vi "TS Station Global Update UI.vi"(8 "error in (no error)":errorcluster, 11 "Auto UI in":refnum<class "Auto UI.lvclass">) -> (0 "error out":errorcluster, 3 "Auto UI out":refnum<class "Auto UI.lvclass">)   [LabVIEW 2023, in "GUI.lvlib" / "Auto UI.lvlib" / "Auto UI.lvclass"]
uses:
  Auto UI.lvclass
  Typdefs/Auto GUI/Test Info.ctl
  Typdefs/Auto GUI/Cycles and Mode.ctl
  Auto UI.lvclass/Auto UI.ctl
  GUI.lvlib
  HardwareAbstractionLayer_LVOOP/Database/Database.lvclass
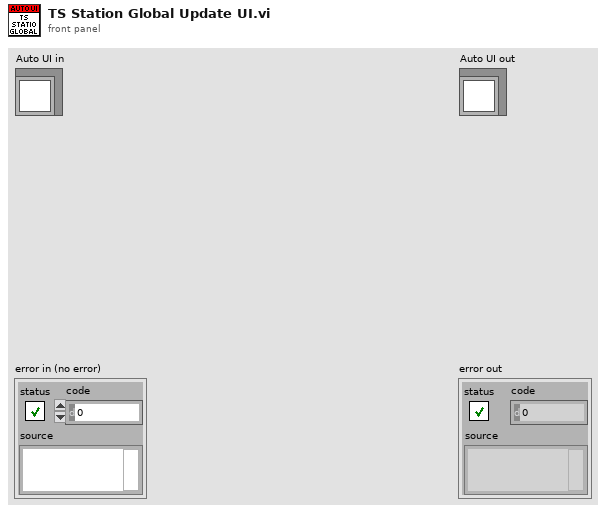
[diagram p1: front panel]
types:
  T1 = cluster{"Total Cycle Number":dbl, "Running Cycle Number":dbl, "Cycle Duration":dbl, "Total Duration":dbl}
  T2 = typedef "GUI.lvlib/Cycles and Mode.ctl" = cluster{"Current Cycle":u32, "Total Cycle":u32, "Current Mode":u32}
  T3 = typedef "GUI.lvlib/Test Info.ctl" = cluster{"Project Name":string, "Product Name":string, "Product Varient":string, "Test Name":string, "Test Start Time":string, "Estimated Date":string}
  T4 = cluster{"Temperature Name":string, "Temperature":i32}
  T5 = cluster{"[0]":i32, "[1]":i32, "[2]":i32, "[3]":i32, "[4]":i32, "[5]":i32}
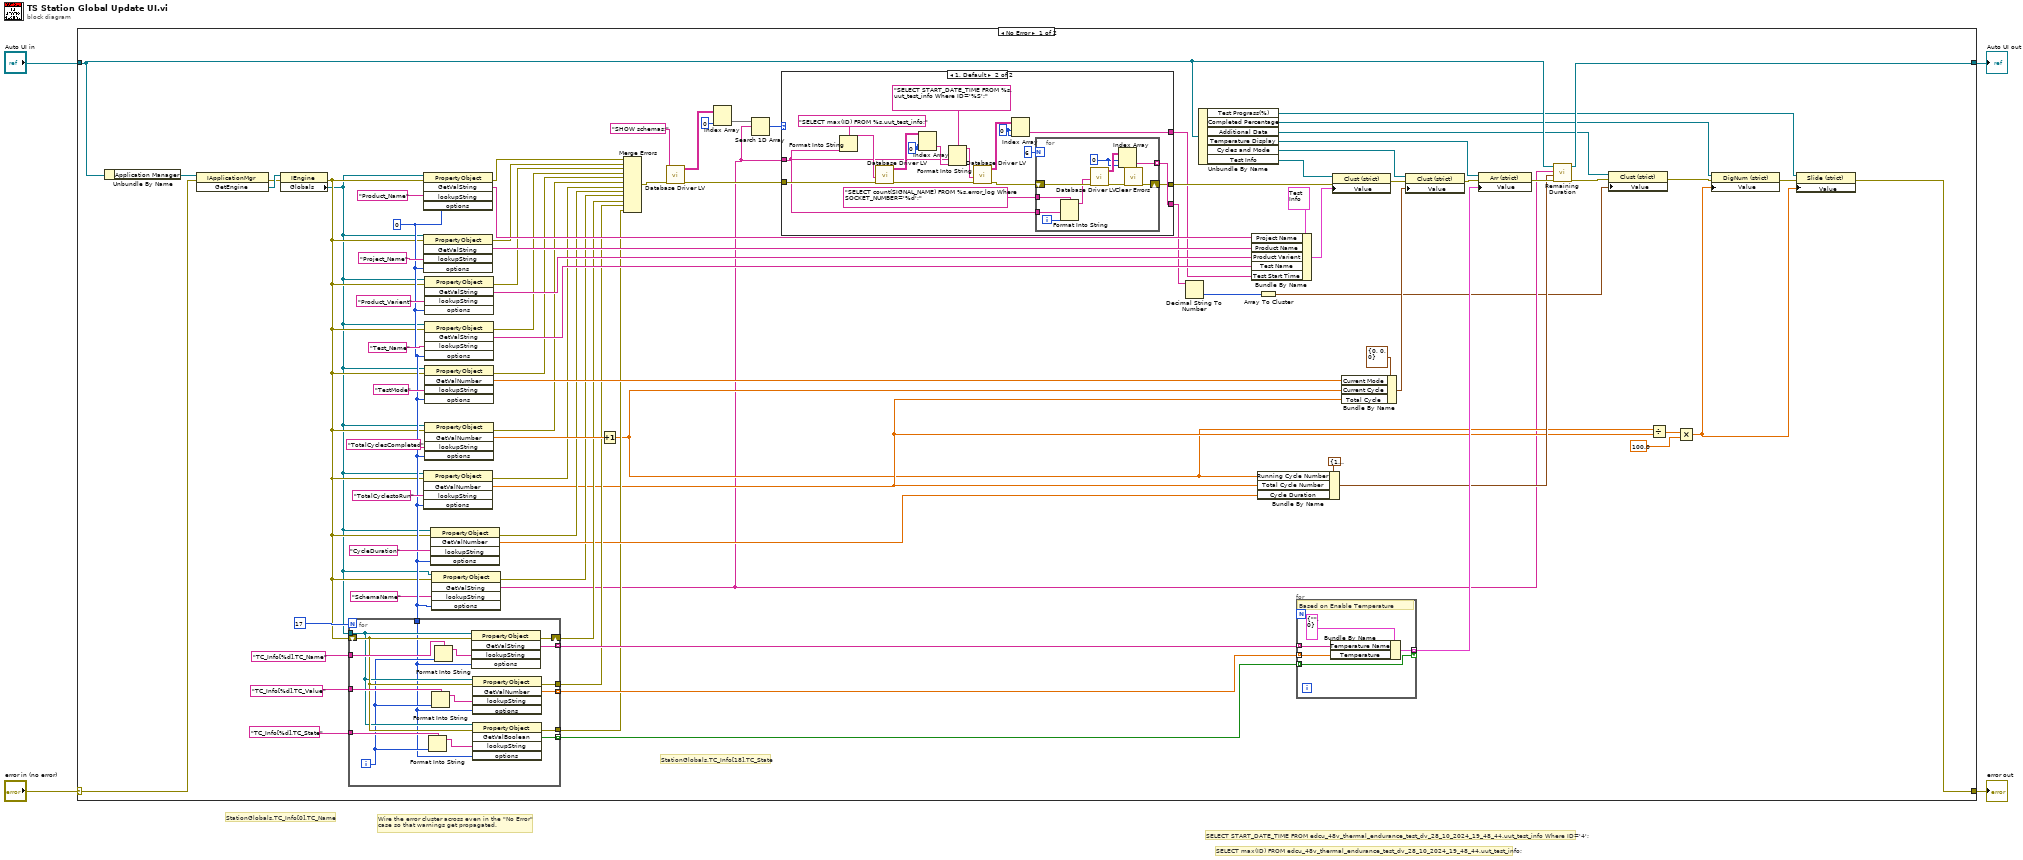
[diagram p0: block diagram]
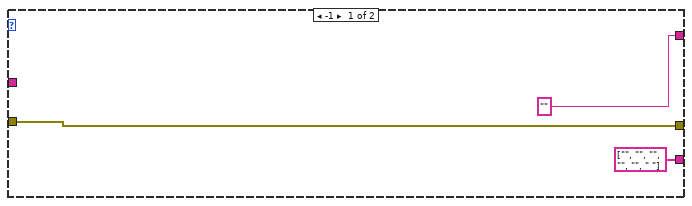
[diagram p2: hidden frame]
diagram:
  # "SELECT max(ID) FROM edcu_48v_thermal_endurance_test_dv_28_10_2024_19_48_44.uut_test_info;"
  # "SELECT START_DATE_TIME FROM edcu_48v_thermal_endurance_test_dv_28_10_2024_19_48_44.uut_test_info Where ID='4';"
  # "StationGlobals.TC_Info[0].TC_Name"
  # "Wire the error cluster across even in the \"No Error\"\ncase so that warnings get propagated."
  n1 = case shown="No Error" "error in (no error)" {
    selector: "error in (no error)" -> [w85 w140]
    tunnel: [w7 w140] -> w3
    tunnel: [w42 w139] -> w1
    tunnel: "Auto UI in" -> [w43 w139]
    frame No Error {
      w37 = 0 ("options")
      # "StationGlobals.TC_Info[18].TC_State"
      n2 = Unbundle By Name(w43) -> ("Application Manager"=w86:refnum<k7>)
      n3 = invoke class="IApplicationMgr" method="GetEngine"(reference=w86, error in=w85) -> (error out=w83:errorcluster, "GetEngine"=w84:refnum<k7>)  [unwired: 1 in, 1 out]
      n4 = property class="IEngine"(reference=w84, error in=w83) -> (error out=w35:errorcluster, "Globals"=w34:refnum<k7>)  [unwired: 1 out]
      n5 = for {
        N: 17 -> [_]
        tunnel: [w133] -> w53 mode=indexing
        tunnel: w37 -> [w118]
        tunnel: w34 -> [w124]
        tunnel: [w131] -> w51
        shift-right: [w132] -> w52
        shift-left: w35 -> [w125]
        tunnel: [w130] -> w50 mode=indexing
        tunnel: "TC_Info[%d].TC_Name" -> [w129]
        tunnel: "TC_Info[%d].TC_Value" -> [w127]
        tunnel: [w123] -> w21
        tunnel: "TC_Info[%d].TC_State" -> [w122]
        tunnel: [w119] -> w22 mode=indexing
        i -> [w121]
        n6 = Format Into String(format string=w122, w121) -> (resulting string=w120:string)  [unwired: 2 in, 1 out]
        n7 = Format Into String(format string=w127, w121) -> (resulting string=w126:string)  [unwired: 2 in, 1 out]
        n8 = Format Into String(format string=w129, w121) -> (resulting string=w128:string)  [unwired: 2 in, 1 out]
        n9 = invoke class="PropertyObject" method="GetValString"(reference=w124, error in=w125, "lookupString"=w128, "options"=w118) -> (error out=w132:errorcluster, "GetValString"=w133:string)  [unwired: 1 in, 3 out]
        n10 = invoke class="PropertyObject" method="GetValNumber"(reference=w124, error in=w125, "lookupString"=w126, "options"=w118) -> (error out=w131:errorcluster, "GetValNumber"=w130:dbl)  [unwired: 1 in, 3 out]
        n11 = invoke class="PropertyObject" method="GetValBoolean"(reference=w124, error in=w125, "lookupString"=w120, "options"=w118) -> (error out=w123:errorcluster, "GetValBoolean"=w119:bool)  [unwired: 1 in, 3 out]
      }
      n12 = invoke class="PropertyObject" method="GetValString"(reference=w34, error in=w35, "lookupString"="Product_Name", "options"=w37) -> (error out=w81:errorcluster, "GetValString"=w77:string)  [unwired: 1 in, 3 out]
      n13 = invoke class="PropertyObject" method="GetValString"(reference=w34, error in=w35, "lookupString"="Project_Name", "options"=w37) -> (error out=w70:errorcluster, "GetValString"=w74:string)  [unwired: 1 in, 3 out]
      n14 = invoke class="PropertyObject" method="GetValNumber"(reference=w34, error in=w35, "lookupString"="TotalCyclestoRun", "options"=w37) -> (error out=w57:errorcluster, "GetValNumber"=w13:dbl)  [unwired: 1 in, 3 out]
      n15 = invoke class="PropertyObject" method="GetValString"(reference=w34, error in=w35, "lookupString"="Product_Varient", "options"=w37) -> (error out=w69:errorcluster, "GetValString"=w71:string)  [unwired: 1 in, 3 out]
      n16 = invoke class="PropertyObject" method="GetValString"(reference=w34, error in=w35, "lookupString"="Test_Name", "options"=w37) -> (error out=w68:errorcluster, "GetValString"=w72:string)  [unwired: 1 in, 3 out]
      n17 = invoke class="PropertyObject" method="GetValNumber"(reference=w34, error in=w35, "lookupString"="TestMode", "options"=w37) -> (error out=w59:errorcluster, "GetValNumber"=w61:dbl)  [unwired: 1 in, 3 out]
      n18 = invoke class="PropertyObject" method="GetValNumber"(reference=w34, error in=w35, "lookupString"="TotalCyclesCompleted", "options"=w37) -> (error out=w58:errorcluster, "GetValNumber"=w60:dbl)  [unwired: 1 in, 3 out]
      n19 = invoke class="PropertyObject" method="GetValNumber"(reference=w34, error in=w35, "lookupString"="CycleDuration", "options"=w37) -> (error out=w45:errorcluster, "GetValNumber"=w39:dbl)  [unwired: 1 in, 3 out]
      n20 = invoke class="PropertyObject" method="GetValString"(reference=w34, error in=w35, "lookupString"="SchemaName", "options"=w37) -> (error out=w33:errorcluster, "GetValString"=w11:string)  [unwired: 1 in, 3 out]
      n21 = Increment(x=w60) -> (x+1=w12:dbl)
      n22 = Merge Errors(w81, w70, w69, w68, w59, w58, w57, w45, w33, w52, w51, w21) -> (w27:errorcluster)
      n23 = call "Database Driver LV.vi"("error in"=w27, "SQL query"="SHOW schemas;") -> ("error out"=w26:errorcluster, "data"=w25:string[][])  [unwired: 6 in, 2 out]
      n24 = Index Array(array=w25, index (col)=0 ("disabled index (col)")) -> (element=w29:string[])  [unwired: 1 in]
      n25 = Search 1D Array(1D array=w29, element=w11) -> (index of element=w28:i32)  [unwired: 1 in]
      n26 = case shown="1, Default" w28 {
        tunnel: w26 -> [w89 w92]
        tunnel: w11 -> [_ w90]
        tunnel: [w89 w93] -> w32
        tunnel: ["" w97] -> w31
        tunnel: [string[] ["", "", "", "", "", " "] w94] -> w18
        frame -1 {
        }
        frame 1, Default {
          w98 = 0 ("index (row)")
          w102 = 0 ("disabled index (col)")
          n27 = Format Into String(format string="SELECT max(ID) FROM %s.uut_test_info;", w90) -> (resulting string=w104:string)  [unwired: 2 in, 1 out]
          n28 = call "Database Driver LV.vi"("error in"=w92, "SQL query"=w104) -> ("error out"=w107:errorcluster, "data"=w103:string[][])  [unwired: 6 in, 2 out]
          n29 = Index Array(array=w103, index (row)=w102, index (col)=w102) -> (element=w101:string)
          n30 = Format Into String(format string="SELECT START_DATE_TIME FROM %s.uut_test_info Where ID='%S';", w90, w101) -> (resulting string=w100:string)  [unwired: 2 in, 1 out]
          n31 = call "Database Driver LV.vi"("error in"=w107, "SQL query"=w100) -> ("error out"=w96:errorcluster, "data"=w99:string[][])  [unwired: 6 in, 2 out]
          n32 = Index Array(array=w99, index (row)=w98, index (col)=w98) -> (element=w97:string)
          n33 = for {
            N: 6 -> [_]
            tunnel: "SELECT count(SIGNAL_NAME) FROM %s.error_log Where SOCKET_NUMBER='%d';" -> [w115]
            tunnel: [w111] -> w94 mode=indexing
            shift-right: [w110] -> w93
            shift-left: w96 -> [w117]
            tunnel: w90 -> [w109]
            i -> [w108]
            w112 = 0 ("index (row)")
            n34 = Format Into String(format string=w115, w109, w108) -> (resulting string=w114:string)  [unwired: 2 in, 1 out]
            n35 = call "Database Driver LV.vi"("error in"=w117, "SQL query"=w114) -> ("error out"=w116:errorcluster, "data"=w113:string[][])  [unwired: 6 in, 2 out]
            n36 = Index Array(array=w113, index (row)=w112, index (col)=w112) -> (element=w111:string)
            n37 = call <vilib>:"Clear Errors.vi"("error in (no error)"=w116) -> ("error out"=w110:errorcluster)  [unwired: 5 in, 1 out]
          }
        }
      }
      n38 = Decimal String To Number(string=w18) -> (number=w6:i32[])  [unwired: 2 in, 1 out]
      n39 = Unbundle By Name(w43) -> ("Test Prograss(%)"=w10:refnum<vi>, "Completed Percentage"=w17:refnum<vi>, "Additional Data"=w20:refnum<vi>, "Temperature Display"=w55:refnum<vi>, "Cycles and Mode"=w64:refnum<vi>, "Test Info"=w80:refnum<vi>)
      n40 = Bundle By Name(cluster=T3 {"Project Name"="ABCD", "Product Name"="ABCD", "Product Varient"="ABCD", "Test Name"="ABCD", "Test Start Time"="ABCD", "Estimated Date"="ABCD"} ("Value"), "Project Name"=w77, "Product Name"=w74, "Product Varient"=w71, "Test Name"=w72, "Test Start Time"=w31) -> (w78:T3)
      n41 = Bundle By Name(cluster=T1 {"Total Cycle Number"=1290.0, "Running Cycle Number"=1.0, "Cycle Duration"=4440.0, "Total Duration"=5727600.0} ("Remain Duration Data"), "Running Cycle Number"=w12, "Total Cycle Number"=w13, "Cycle Duration"=w39) -> (w38:T1)
      n42 = Array To Cluster(array=w6) -> (cluster=w5:T5)
      n43 = for {
        tunnel: [w138] -> w54 mode=indexing if=w134
        tunnel: w53 -> [w137] mode=indexing
        tunnel: w50 -> [w136] mode=indexing
        tunnel: w22 -> [w134] mode=indexing
        # "Based on Enable Temperature"
        n44 = Bundle By Name(cluster=T4 {"Temperature Name"="", "Temperature"=0} ("Temperature"), "Temperature Name"=w137, "Temperature"=w136) -> (w138:T4)
      }
      n45 = property class="Clust (strict)"(reference=w80, error in=w32, "Value"=w78) -> (error out=w63:errorcluster)  [unwired: 1 out]
      n46 = Bundle By Name(cluster=T2 {"Current Cycle"=0, "Total Cycle"=0, "Current Mode"=0} ("Value"), "Current Mode"=w61, "Current Cycle"=w12, "Total Cycle"=w13) -> (w56:T2)
      n47 = property class="Clust (strict)"(reference=w64, error in=w63, "Value"=w56) -> (error out=w44:errorcluster)  [unwired: 1 out]
      n48 = property class="Arr (strict)"(reference=w55, error in=w44, "Value"=w54) -> (error out=w41:errorcluster)  [unwired: 1 out]
      n49 = call "Remaining Duration.vi"("error in (no error)"=w41, "Remain Duration Data"=w38, "Schema"=w11, "Auto UI in"=w43) -> ("error out"=w19:errorcluster, "Auto UI out"=w42:refnum<class "Auto UI.lvclass">)  [unwired: 6 in]
      n50 = property class="Clust (strict)"(reference=w20, error in=w19, "Value"=w5) -> (error out=w16:errorcluster)  [unwired: 1 out]
      n51 = Divide(x=w12, y=w13) -> (x/y=w15:dbl)
      n52 = Multiply(x=w15, y=100.0) -> (x*y=w9:dbl)
      n53 = property class="DigNum (strict)"(reference=w17, error in=w16, "Value"=w9) -> (error out=w8:errorcluster)  [unwired: 1 out]
      n54 = property class="Slide (strict)"(reference=w10, error in=w8, "Value"=w9) -> (error out=w7:errorcluster)  [unwired: 1 out]
    }
    frame Error {
    }
  }
  "error out" <- w3
  "Auto UI out" <- w1
